vi "IDS_ecu_getTemperatureInDegrees.vi"(0 "deviceHandle":i32, 1 "error in (no error)":errorcluster) -> (2 "deviceHandle out":i32, 3 "temp out":dbl, 4 "error out":errorcluster)   [LabVIEW 2016]
doc: "int IDS_DLL IDS_ecu_enable();"
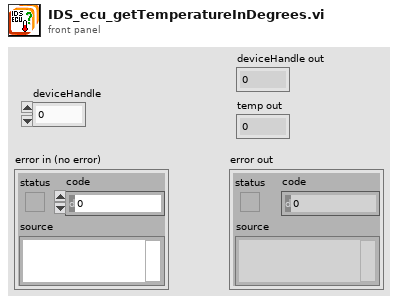
[diagram p1: front panel]
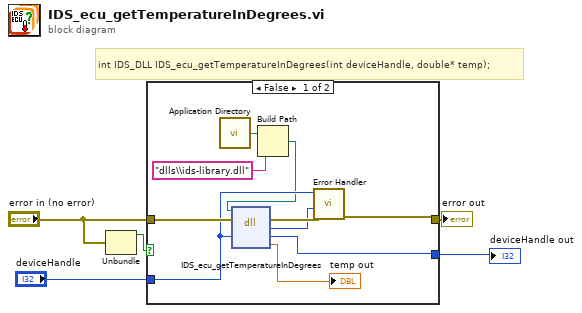
[diagram p0: block diagram]
diagram:
  # "int IDS_DLL IDS_ecu_getTemperatureInDegrees(int deviceHandle, double* temp);"
  n1 = Unbundle("error in (no error)") -> ("status"=w1:bool)  [unwired: 2 out]
  n2 = case shown="False" w1 {
    tunnel: "error in (no error)" -> [w15 w17]
    tunnel: [w13 w17] -> w5
    tunnel: "deviceHandle" -> [w11 w16]
    tunnel: [w12 w16] -> w3
    frame False {
      n3 = call <vilib>:"Application Directory.vi"() -> ("Application Directory"=w8:path)
      n4 = Build Path(base path=w8, name or relative path="dlls\\ids-library.dll" ("ipAddress")) -> (appended path=w6:path)
      n5 = dll-call lib="C:/Users/matheus/Desktop/LabVIEW_Draft_V1.6.0/dlls/ids-library.*" fn="IDS_ecu_getTemperatureInDegrees"(path in=w6, error in=w15, "deviceHandle"=w11) -> (error out=w14:errorcluster, "return type"=w10:i32, "deviceHandle"=w12:i32, "temp"=→"temp out":dbl)  [unwired: 2 in, 1 out]
      n6 = call "Error Handler.vi"("error in (no error)"=w14, "error code"=w10, "deviceHandle"=w11) -> ("error out"=w13:errorcluster)  [unwired: 7 in, 1 out]
    }
    frame True {
    }
  }
  "error out" <- w5
  "deviceHandle out" <- w3
